vi "TX ADU.vi"(8 "error in (no error)":errorcluster, 9 "PDU_req in":T1={"Function Code"=1, "Data"=[], "RTU_DataBytes"=0}, 10 "VISA resource in":refnum<visa-resource-name>, 11 "MB_ADU in":refnum<class "MB_ADU_Serial.lvclass">) -> (0 "error out":errorcluster, 1 "PDU_req out":T1={"Function Code"=1, "Data"=[], "RTU_DataBytes"=0}, 2 "VISA resource out":refnum<visa-resource-name>, 3 "MB_ADU out":refnum<class "MB_ADU_Serial.lvclass">)   [LabVIEW 2023, in "Jiaxin_Stepper_Controller.lvlib" / "MB Master.lvlib" / "MB_ADU_Serial.lvclass"]
doc: "Defines the Modbus transmit ADU process. This is specific to the mode (RTU or ASCII)."
uses:
  MB_ADU_Serial.lvclass
  MB_PDU/MB_PDU_Cluster.ctl
  MB Master.lvlib
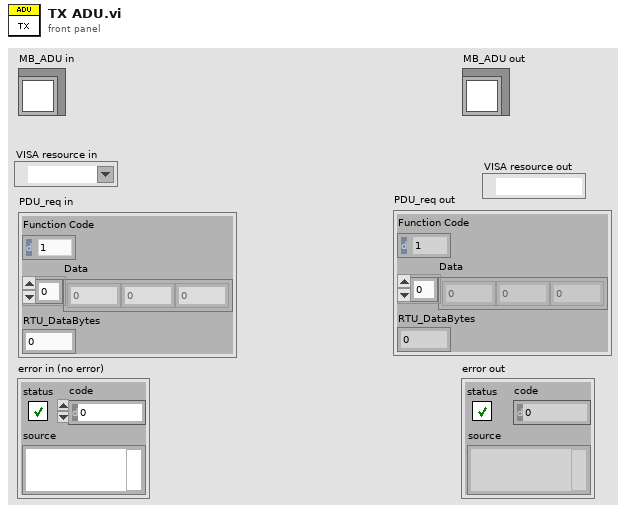
[diagram p1: front panel]
types:
  T1 = typedef "Jiaxin_Stepper_Controller.lvlib/MB Master.lvlib/MB_PDU_Cluster.ctl" = cluster{"Function Code":u8, "Data":u8[], "RTU_DataBytes":i32}
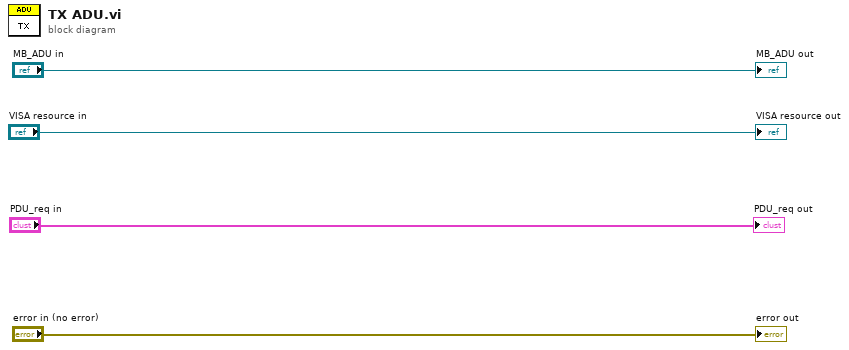
[diagram p0: block diagram]
diagram:
  "error out" <- "error in (no error)"
  "MB_ADU out" <- "MB_ADU in"
  "VISA resource out" <- "VISA resource in"
  "PDU_req out" <- "PDU_req in"
